vi "Get Item Value From Properties by Name.vi"(8 "error in (no error)":errorcluster caption="错误输入（无错误）", 9 "Enable":bool=TRUE, 10 "PropertyName":string, 11 "ManagementClass 输入":refnum<class "ManagementClass.lvclass"> caption="DNL_LabVIEW Object in") -> (0 "error out":errorcluster caption="错误输出", 2 "Value":string, 3 "ManagementClass 输出":refnum<class "ManagementClass.lvclass"> caption="DNL_LabVIEW Object out")   [LabVIEW 2013, in "ManagementClass.lvclass"]
uses:
  ManagementClass.lvclass
  ManagementClass.lvclass/ManagementClass.ctl
  System.Management
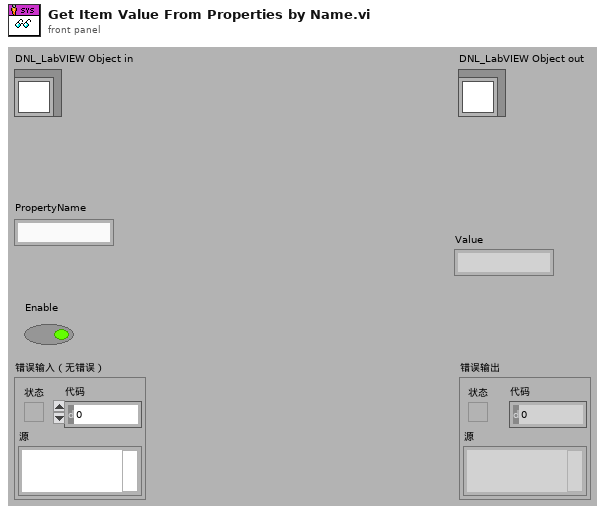
[diagram p1: front panel]
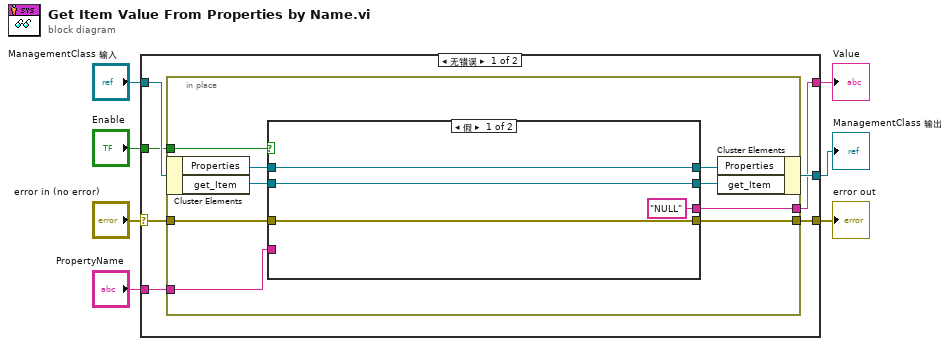
[diagram p0: block diagram]
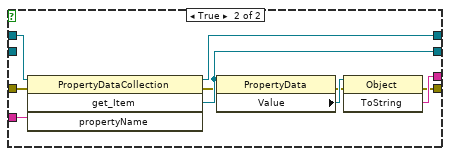
[diagram p2: hidden frame]
diagram:
  n1 = case shown="无错误" "error in (no error)" {
    selector: "error in (no error)" -> [w12 w39]
    tunnel: [w9 w39] -> w6
    tunnel: [w13 w38] -> w4
    tunnel: "ManagementClass 输入" -> [w14 w38]
    tunnel: [w11 _] -> w3
    tunnel: "PropertyName" -> [w10 _]
    tunnel: "Enable" -> [w8 _]
    frame No Error {
      n2 = in-place {
        in-place-border: w12 -> [w20]
        in-place-border: [w19] -> w11
        in-place-border: w10 -> [w18]
        in-place-border: [w17] -> w9
        in-place-border: w8 -> [w16]
        n3 = in-place-cluster #1(w14) -> ("Properties"=w23:refnum<k24>, "get_Item"=w15:refnum<k24>)
        n4 = case shown="假" w16 {
          tunnel: w23 -> [w27 w37]
          tunnel: [w27 w35] -> w22
          tunnel: [w26 w34] -> w21
          tunnel: w20 -> [w25 w33]
          tunnel: ["NULL" ("ToString") w32] -> w19
          tunnel: w18 -> [_ w31]
          tunnel: [w25 w28] -> w17
          tunnel: w15 -> [w26 _]
          frame False {
          }
          frame True {
            n5 = invoke class="PropertyDataCollection" method="get_Item"(reference=w37, error in=w33, "propertyName"=w31) -> (reference out=w35:refnum<k24>, error out=w30:errorcluster, "get_Item"=w34:refnum<k24>)  [unwired: 1 in, 1 out]
            n6 = property class="PropertyData"(reference=w34, error in=w30) -> (error out=w29:errorcluster, "Value"=w36:refnum<k24>)  [unwired: 1 out]
            n7 = invoke class="Object" method="ToString"(reference=w36, error in=w29) -> (error out=w28:errorcluster, "ToString"=w32:string)  [unwired: 1 in, 1 out]
          }
        }
        n8 = in-place-cluster #1("Properties"=w22, "get_Item"=w21) -> (w13:refnum<class "ManagementClass.lvclass">)
      }
    }
    frame Error {
    }
  }
  "error out" <- w6
  "ManagementClass 输出" <- w4
  "Value" <- w3
